vi "Test Deserialize Null.vi"(8 "error in (no error)":errorcluster) -> (0 "error out":errorcluster)   [LabVIEW 2013]
uses:
  <vilib>/addons/_JKI Toolkits/Caraya/classes/Test/Test.lvclass
  src/JKI JSON Serialization.lvlib
  <vilib>/addons/_JKI Toolkits/Caraya/classes/Assert/Assert.lvclass
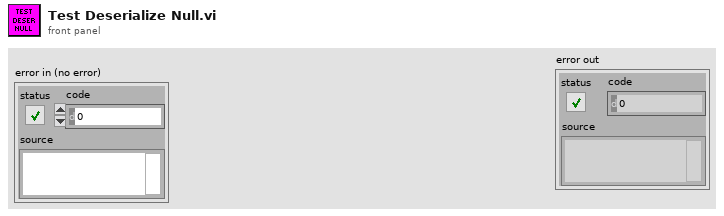
[diagram p1: front panel]
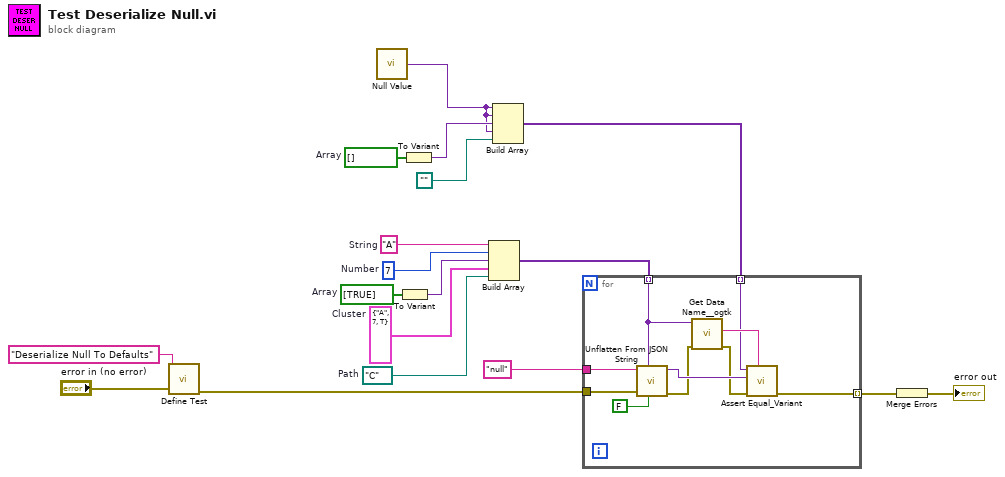
[diagram p0: block diagram]
diagram:
  w3 = path "C:/"  # Path
  w6 = bool[] []  # Array
  w9 = cluster{"String":string, "Number":i32, bool} {"String"="A", "Number"=7, TRUE}  # Cluster
  w10 = bool[] [TRUE]  # Array
  w11 = 7  # Number
  w7 = "A"  # String
  n1 = call <vilib>:"Define Test.vi"("error in (no error)"="error in (no error)", "Label (VI Title)"="Deserialize Null To Defaults") -> ("error out"=w13:errorcluster)  [unwired: 9 in]
  n2 = call "Null Value.vi"() -> ("Null"=w4:variant)
  n3 = To Variant(anything=w10) -> (Variant=w8:variant)
  n4 = To Variant(anything=w6) -> (Variant=w5:variant)
  n5 = Build Array(w7, w11, w8, w9, w3) -> (w12:variant[])
  n6 = Build Array(w4, w4, w5, w4, path "") -> (w1:variant[])
  n7 = for {
    tunnel: "null" ("JSON String") -> [w28]
    tunnel: [w22] -> w14 mode=indexing
    tunnel: w13 -> [w21]
    tunnel: w12 -> [w20] mode=indexing
    tunnel: w1 -> [w19] mode=indexing
    n8 = call "Unflatten From JSON String.vi"("Nulls as Defaults (T)"=FALSE, "Type and Defaults"=w20, "error in (no error)"=w21, "JSON String"=w28) -> ("error out"=w24:errorcluster, "Variant"=w26:variant)  [unwired: 6 in]
    n9 = call <userlib>:"Get Data Name__ogtk.vi"("error in (no error)"=w24, "Data"=w20) -> ("error out"=w23:errorcluster, "Data Name"=w25:string)  [unwired: 7 in, 1 out]
    n10 = call <vilib>:"Assert Equal_Variant.vi"("Label"=w25, "error in (no error)"=w23, "Y"=w26, "X"=w19) -> ("error out"=w22:errorcluster)  [unwired: 7 in]
  }
  n11 = Merge Errors(w14) -> (→"error out":errorcluster)
